vi "PopulateExposureResolution.vi"(10 "Exposure Resolution":refnum<vi>, 11 ".NET Refnum in":refnum<k24>) -> ()   [LabVIEW 2018]
uses:
  D:/SVN/PM/sdk/AppSamples/LabVIEWSamples/trunk/Release/2018/Dependencies/PVCamNET.dll
  Dependencies/PVCamNET.dll
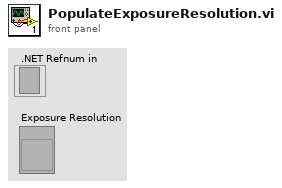
[diagram p1: front panel]
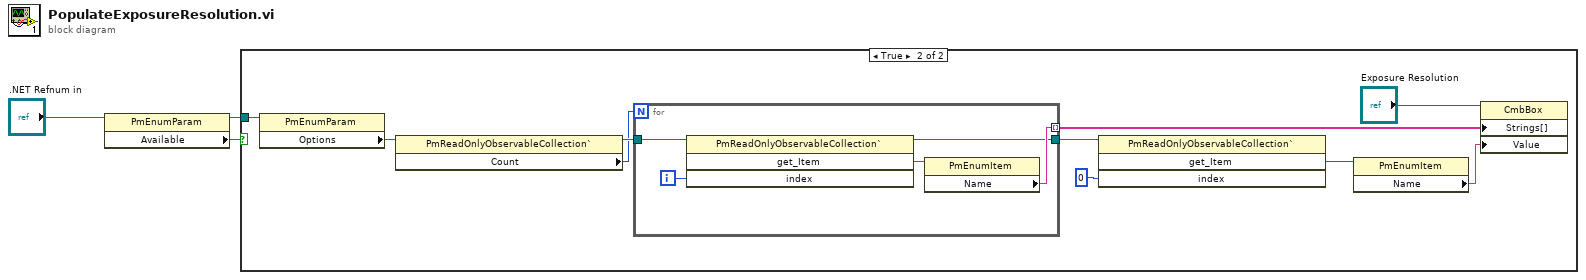
[diagram p0: block diagram]
diagram:
  n1 = property class="PmEnumParam"(reference=".NET Refnum in") -> (reference out=w3:refnum<k24>, "Available"=w1:bool)  [unwired: 1 in, 1 out]
  n2 = case shown="True" w1 {
    tunnel: w3 -> [_ w4]
    frame False {
    }
    frame True {
      n3 = property class="PmEnumParam"(reference=w4) -> ("Options"=w5:refnum<k24>)  [unwired: 1 in, 2 out]
      n4 = property class="PmReadOnlyObservableCollection`"(reference=w5) -> (reference out=w7:refnum<k24>, "Count"=w6:i32)  [unwired: 1 in, 1 out]
      n5 = for {
        N: w6 -> [_]
        tunnel: w7 -> [w18]
        tunnel: [w15] -> w13 mode=indexing
        tunnel: [w14] -> w8
        i -> [w17]
        n6 = invoke class="PmReadOnlyObservableCollection`" method="get_Item"(reference=w18, "index"=w17) -> (reference out=w14:refnum<k24>, "get_Item"=w16:refnum<k24>)  [unwired: 2 in, 2 out]
        n7 = property class="PmEnumItem"(reference=w16) -> ("Name"=w15:string)  [unwired: 1 in, 2 out]
      }
      n8 = invoke class="PmReadOnlyObservableCollection`" method="get_Item"(reference=w8, "index"=0) -> ("get_Item"=w10:refnum<k24>)  [unwired: 2 in, 3 out]
      n9 = property class="PmEnumItem"(reference=w10) -> ("Name"=w12:string)  [unwired: 1 in, 2 out]
      n10 = property class="CmbBox"(reference="Exposure Resolution", "Strings[]"=w13, "Value"=w12) -> ()  [unwired: 1 in, 2 out]
    }
  }
